vi "ModifyMyClassAttribute.vi"(1 "string":string, 5 "error in (no error)":errorcluster) -> (19 "error out":errorcluster)   [LabVIEW 2017, in "MyOrdinaryClass.lvclass"]
uses:
  MyOrdinaryClass.lvclass
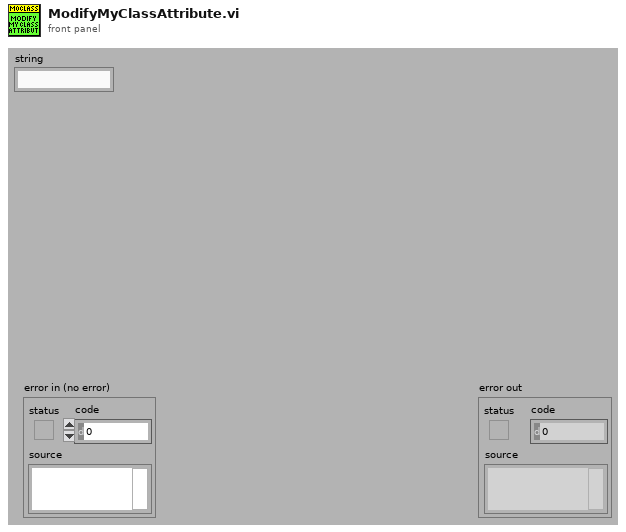
[diagram p1: front panel]
types:
  T1 = typedef "MyOrdinaryClass.lvclass/ClassAttributesRef.ctl" = refnum<data-value>
  T2 = typedef "MyOrdinaryClass.lvclass/ClassAttributes.ctl" = cluster{"MyClassAttribute":string}
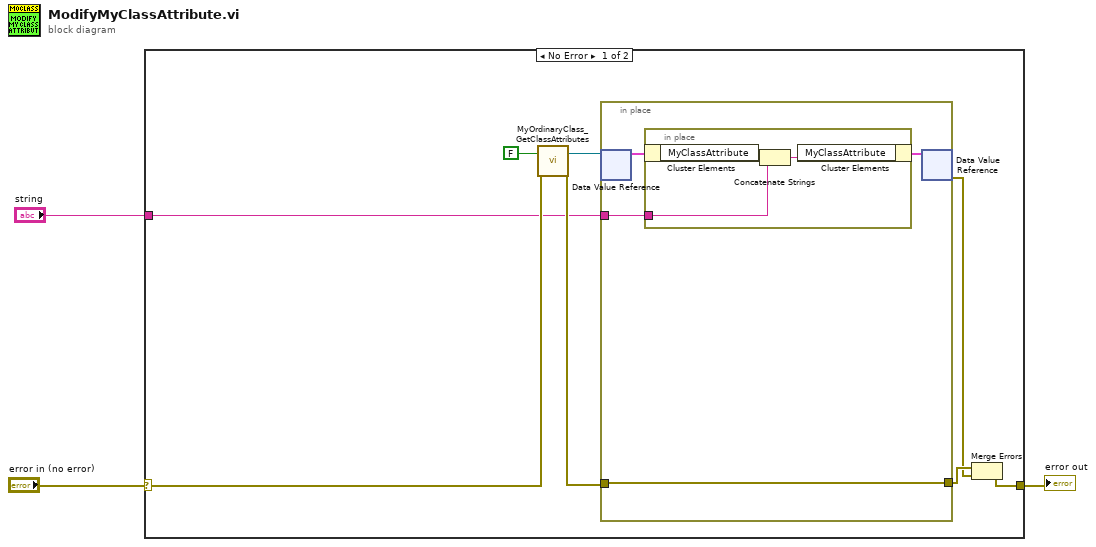
[diagram p0: block diagram]
diagram:
  n1 = case shown="No Error" "error in (no error)" {
    selector: "error in (no error)" -> [w11 w19]
    tunnel: [w8 w19] -> w2
    tunnel: "string" -> [w4 _]
    frame No Error {
      n2 = call "MyOrdinaryClass_GetClassAttributes.vi"("return data? (T)"=FALSE ("return data"), "error in (no error)"=w11) -> ("class attributes ref"=w9:T1, "error out"=w10:errorcluster)  [unwired: 14 in, 2 out]
      n3 = in-place {
        in-place-border: w10 -> [w13]
        in-place-border: [w13] -> w6
        in-place-border: w4 -> [w12]
        n4 = in-place-dvr #1(w9) -> (w14:T2)  [unwired: 1 out]
        n5 = in-place {
          in-place-border: w12 -> [w16]
          n6 = in-place-cluster #2(w14) -> ("MyClassAttribute"=w18:string)
          n7 = Concatenate Strings(w18, w16) -> (w17:string)
          n8 = in-place-cluster #2("MyClassAttribute"=w17) -> (w15:T2)
        }
        n9 = in-place-dvr #1(w15) -> (w5:errorcluster)  [unwired: 1 out]
      }
      n10 = Merge Errors(w6, w5) -> (w8:errorcluster)
    }
    frame Error {
    }
  }
  "error out" <- w2
